vi "test Get Attribute as DBL3.vi"(11 "Test Case In":refnum<class "Test Config From Excel Table.lvclass">) -> (0 "error out":errorcluster, 3 "Test Case Out":refnum<class "Test Config From Excel Table.lvclass">)   [LabVIEW 2020, in "Test Config From Excel Table.lvclass"]
uses:
  Test Config From Excel Table.lvclass
  C:/Program Files/National Instruments/LabVIEW 2025/vi.lib/Astemes/LUnit/Test Case.lvclass
  Source/Config from Excel Table/Config from Excel Table.lvclass
  <vilib>/Astemes/LUnit/Test Case.lvclass/Test Case.ctl
  <vilib>/Astemes/LUnit/Test Case.lvclass
  <vilib>/Peter/Open Xml/Source/Open Xml.lvlib
  4721e792-12f6-44ed-8f8f-b4c64d477831.vi
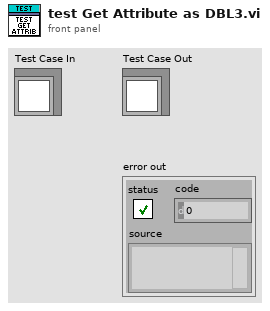
[diagram p1: front panel]
types:
  T1 = cluster{"Sheet Name":string, "Name":string, "Display Name":string, "Range or Cell Address":string}
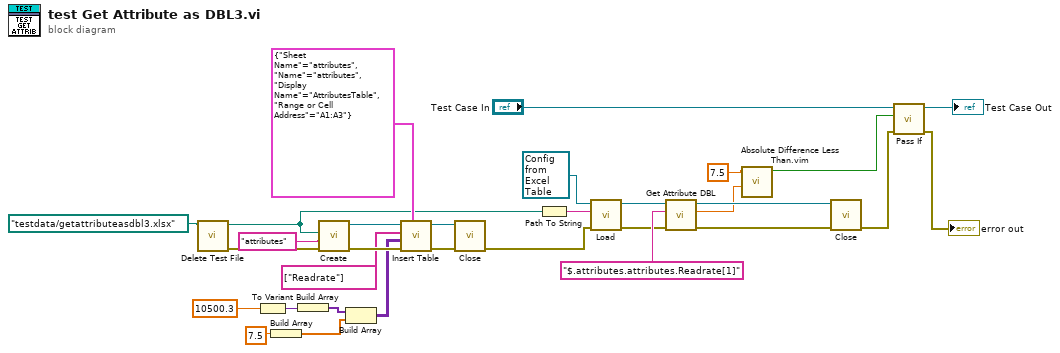
[diagram p0: block diagram]
diagram:
  n1 = call "Delete Test File.vi"("name or relative path"=path "testdata/getattributeasdbl3.xlsx") -> ("error out"=w20:errorcluster, "deleted path"=w8:path)  [unwired: 9 in]
  n2 = To Variant(anything=10500.3) -> (Variant=w14:variant)
  n3 = Build Array(7.5) -> (w4:dbl[])
  n4 = Build Array(w14) -> (w13:variant[])
  n5 = call <vilib>:"Create.vi"("error in"=w20, "SheetName"="attributes", "Path"=w8) -> ("error out"=w19:errorcluster, "SpreadsheetDoc"=w11:refnum<k24>)  [unwired: 7 in]
  n6 = Build Array(w13, w4) -> (w12:variant[][])
  n7 = call <vilib>:"Insert Table.vi"("Location"=T1 {"Sheet Name"="attributes", "Name"="attributes", "Display Name"="AttributesTable", "Range or Cell Address"="A1:A3"}, "error in"=w19, "Cell Values"=w12, "Header Names"=string[] ["Readrate"], "SpreadsheetDoc in"=w11) -> ("error out"=w18:errorcluster, "SpreadsheetDoc out"=w9:refnum<k24>)  [unwired: 5 in]
  n8 = call <vilib>:"Close.vi"("error in"=w18, "SpreadsheetDoc"=w9) -> ("error out"=w10:errorcluster)  [unwired: 9 in]
  n9 = Path To String(path=w8) -> (string=w27:string)
  n10 = call-dynamic "Load.vi"("error in"=w10, "Source"=w27, "Config from Excel Table in"=refnum<class "Config from Excel Table.lvclass"> refnum ("Config from EXCEL Table.lvclass")) -> ("error out"=w21:errorcluster, "Config from Excel Table out"=w22:refnum<class "Config from Excel Table.lvclass">)  [unwired: 7 in]
  n11 = call-dynamic "Get Attribute DBL.vi"("error in"=w21, "Attribute"="$.attributes.attributes.Readrate[1]", "Config from Excel Table in"=w22) -> ("error out"=w24:errorcluster, "Value"=w1:dbl, "Config from Excel Table out"=w25:refnum<class "Config from Excel Table.lvclass">)  [unwired: 6 in]
  n12 = call "Absolute Difference Less Than.vim"("Number 2"=w1, "Number 1"=7.5 ("Value")) -> ("In Limit"=w2:bool)  [unwired: 9 in]
  n13 = call-dynamic <vilib>:"Close.vi"("error in"=w24, "Config from Excel Table in"=w25) -> ("error out"=w23:errorcluster)  [unwired: 8 in, 1 out]
  n14 = call <vilib>:"Pass If.vi"("error in (no error)"=w23, "Pass?"=w2, "LUnit Test Case In"="Test Case In") -> ("error out"=→"error out":errorcluster, "LUnit Test Case Out"=→"Test Case Out":refnum<class "Test Config From Excel Table.lvclass">)  [unwired: 7 in]
